vi "Time_Converter.vi"(0 "Stop_Watch_Time":dbl caption="Stop Watch Time") -> (4 "Time_Format":T1 caption="Time Format")   [LabVIEW 2021]
uses:
  Controls/Time_Format.ctl
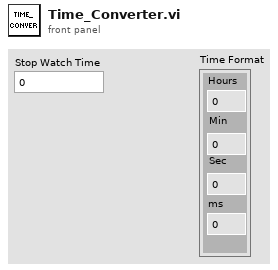
[diagram p1: front panel]
types:
  T1 = typedef "Time_Format.ctl" = cluster{"Hours":i32, "Min":i32, "Sec":i32, "ms":i32}
  T2 = typedef "LVDateTimeRec.ctl" = cluster{"fractional second":dbl, "second":i32, "minute":i32, "hour":i32, "day of month":i32, "month":i32, "year":i32, "day of week":i32, "day of year":i32, "DST":i32}
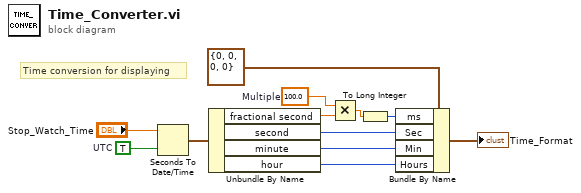
[diagram p0: block diagram]
diagram:
  w4 = 100.0  # Multiple
  w8 = TRUE  # UTC
  # "Time conversion for displaying"
  n1 = Seconds To Date/Time(time stamp (now)="Stop_Watch_Time", to UTC (F)=w8) -> (date time rec=w12:T2)
  n2 = Unbundle By Name(w12) -> ("fractional second"=w6:dbl, "second"=w10:i32, "minute"=w11:i32, "hour"=w1:i32)
  n3 = Multiply(x=w4, y=w6) -> (x*y=w5:dbl)
  n4 = To Long Integer(number=w5) -> (32bit integer=w3:i32)
  n5 = Bundle By Name(cluster=T1 {"Hours"=0, "Min"=0, "Sec"=0, "ms"=0} ("Cluster 3"), "ms"=w3, "Sec"=w10, "Min"=w11, "Hours"=w1) -> (→"Time_Format":T1)
